vi "01_Übertragungsfunktion.vi"() -> ()   [LabVIEW 2019]
uses:
  <vilib>/Analysis/2dsp.llb/Real FFT.vi
  <vilib>/Analysis/NI_AALPro.lvlib
panel:
  out "Phase":dbl[](graph)
  out "Amplitude":dbl[](graph)
  out "Imaginärteil":dbl[](graph)
  out "Realteil":dbl[](graph)
  out "accel":dynamicdata(graph) caption="data"
  out "force":dynamicdata(graph) caption="data"
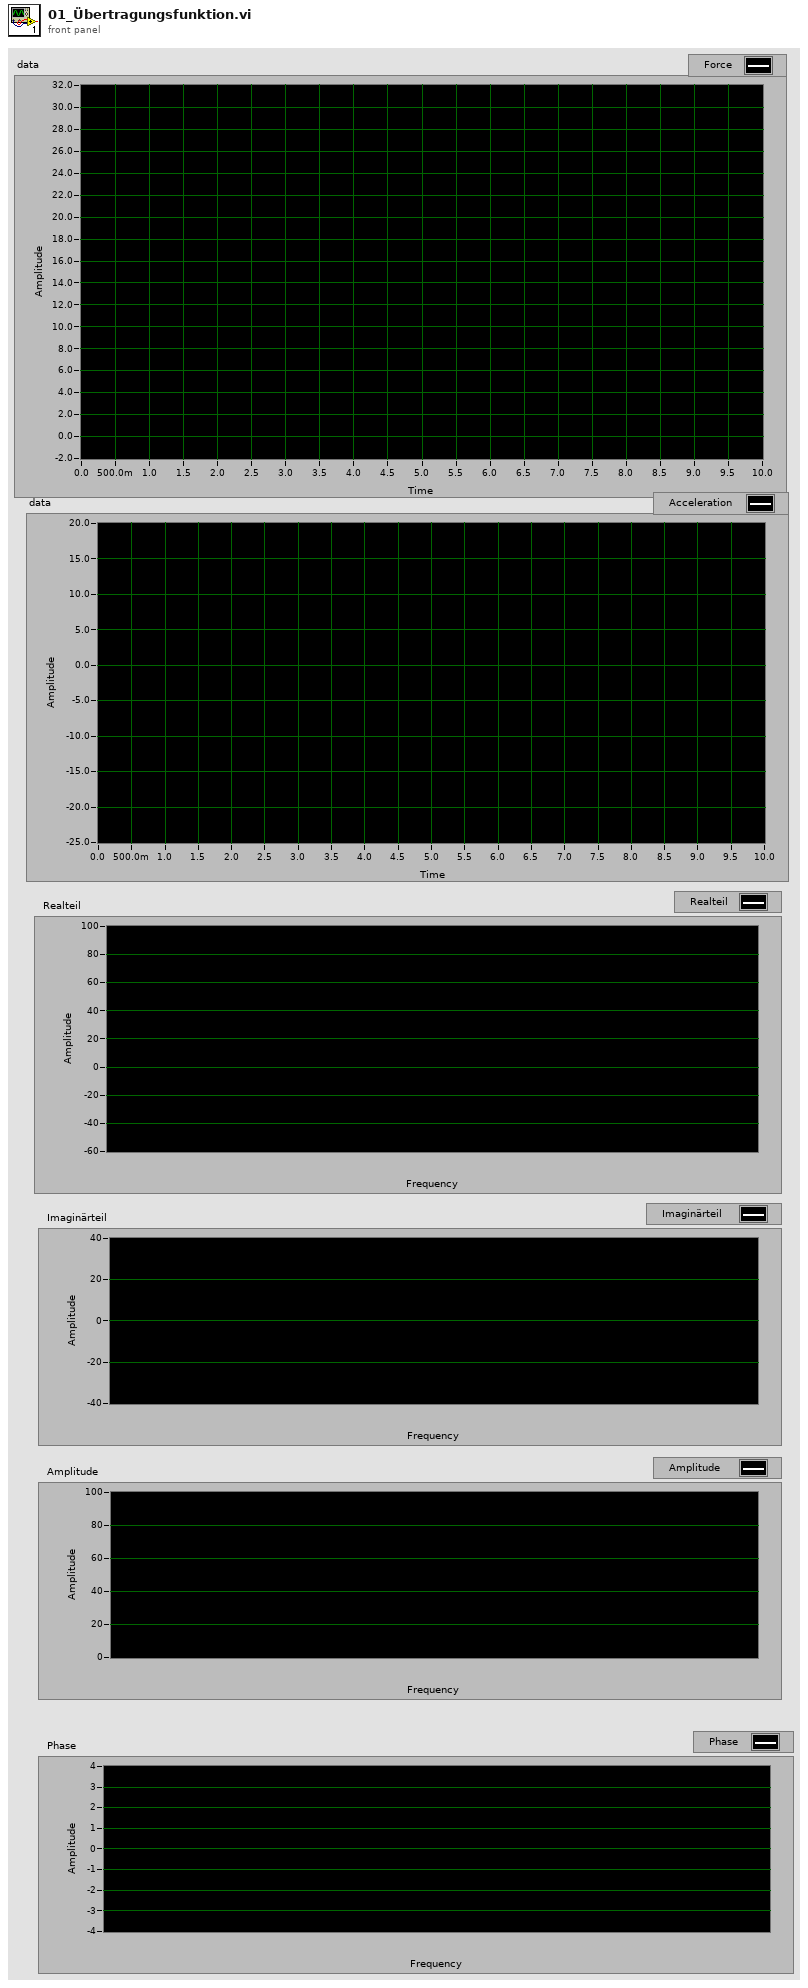
[diagram p1: front panel]
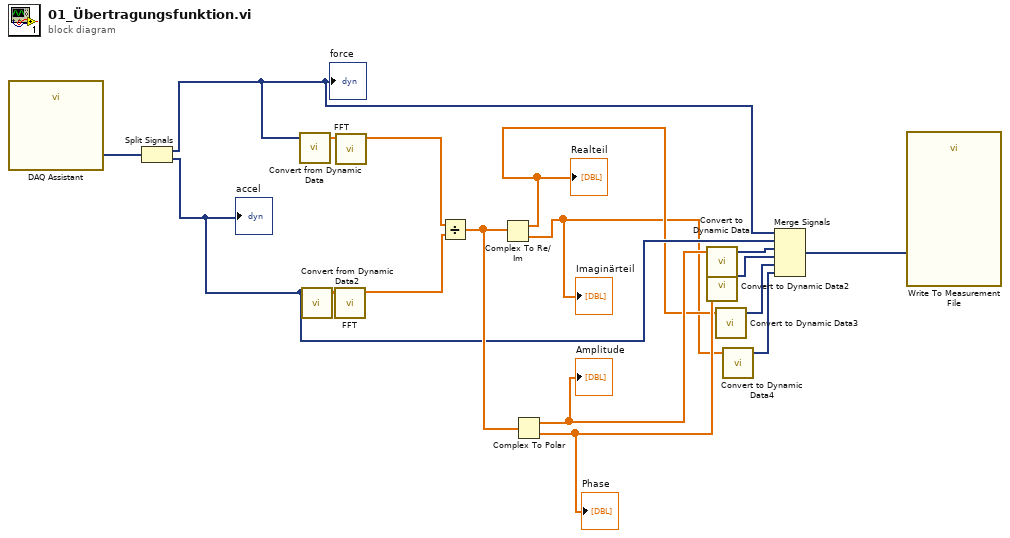
[diagram p0: block diagram]
diagram:
  n1 = call "DAQ Assistant"() -> ("data"=w17:dynamicdata)  [unwired: 17 in, 2 out]
  n2 = Split Signals(w17) -> (w11:dynamicdata, w10:dynamicdata)  [unwired: 2 in]
  "force" <- w11
  "accel" <- w10
  n3 = call "Convert from Dynamic Data"("Dynamic Data Type"=w11) -> ("Array"=w16:dbl[])  [unwired: 3 in]
  n4 = call "Convert from Dynamic Data2"("Dynamic Data Type"=w10) -> ("Array"=w15:dbl[])  [unwired: 3 in]
  n5 = call-poly <vilib>:"FFT.vi"("X"=w15) -> ("FFT {X}"=w13:cdb[])  [unwired: 9 in, 1 out]
  n6 = call-poly <vilib>:"FFT.vi"("X"=w16) -> ("FFT {X}"=w14:cdb[])  [unwired: 9 in, 1 out]
  n7 = Divide(x=w14, y=w13) -> (x/y=w12:cdb[])
  n8 = Complex To Re/Im(x + iy=w12) -> (x=w4:dbl[], y=w2:dbl[])
  "Realteil" <- w4
  "Imaginärteil" <- w2
  n9 = Complex To Polar(r * e^(i*theta)=w12) -> (r=w5:dbl[], theta=w7:dbl[])
  "Amplitude" <- w5
  "Phase" <- w7
  n10 = call "Convert to Dynamic Data"("Array"=w5) -> ("Dynamic Data Type"=w9:dynamicdata)  [unwired: 3 in]
  n11 = call "Convert to Dynamic Data2"("Array"=w7) -> ("Dynamic Data Type"=w6:dynamicdata)  [unwired: 3 in]
  n12 = call "Convert to Dynamic Data3"("Array"=w4) -> ("Dynamic Data Type"=w3:dynamicdata)  [unwired: 3 in]
  n13 = call "Convert to Dynamic Data4"("Array"=w2) -> ("Dynamic Data Type"=w1:dynamicdata)  [unwired: 3 in]
  n14 = Merge Signals(w11, w10, w9, w6, w3, w1) -> (w8:dynamicdata)
  n15 = call "Write To Measurement File"("Signals"=w8) -> ()  [unwired: 16 in, 3 out]
